vi "TLB Native Dynamic Events ver 0.07c.vi"() -> ()   [LabVIEW 2018]
uses:
  Labview Training Phase 2/Enum Controls/States for Action Engine.ctl
  Type def/TLB event states.ctl
  Type def/TLB MHL States.ctl
  <vilib>/Studica/Studica Toolkit/Background/I2C Channel.ctl
  <vilib>/Studica/Studica Toolkit/NavX/NavX.lvlib
  <vilib>/myRIO/Common/Instrument Driver Framework/myRIO v1.0/AI/typedefs/AI Channels Enum.ctl
  <vilib>/myRIO/Common/Instrument Driver Framework/myRIO v1.0/AI/typedefs/AI Channels List.ctl
  Type def/Type def.ctl
  Type def/Motor Control Cluster.ctl
  <vilib>/Studica/Studica Blackhawk/Blackhawk.lvlib
  <vilib>/Studica/Studica Toolkit/Background/Mxp Selection.ctl
  <vilib>/Studica/Studica Toolkit/Background/DIO Channel.ctl
  <vilib>/NI_Real-Time Target Support.lvlib
  <vilib>/ptbypt/NI_PtbyPt.lvlib
  <vilib>/addons/control/pid/NI_PID_pid.lvlib
  <vilib>/addons/control/pid/pid.llb/PID (DBL).vi
  Underlying VI's/Webcam FGV Low level ver/State control.ctl
  <vilib>/userdefined/High Color/IMAQdx.ctl
panel:
  out "Manual Zero Yaw":bool
  out "Cluster":T1
  out "Displacement":T2
  out "Fused Heading":dbl
  in  "error in (no error)":errorcluster
  in  "RED LED State":enum16{"OFF", "ON", "BLINK"}(ring)
  in  "GREEN LED State":enum16{"OFF", "ON", "BLINK"}(ring)
  in  "Red LED":bool
  in  "Green LED":bool
  in  "NavX Zero Yaw":bool
  out "Input state":i8
  out "Waveform Chart 2":dbl(graph)
  out "Waveform Chart":dbl(graph)
  in  "STOP":bool
  out "DIO 0":bool
  out "DIO 1":bool
  out "Limit Switch Array":bool[](array[boolean])
  out "error out":errorcluster
  out "L/R average":fxp<+,64,64>
  out "Right Ultrasonic":fxp<+,64,16>
  out "Left Ultrasonic":fxp<+,64,16>
  out "Right IR Sensor":dbl
  out "Left IR Sensor":dbl
  out "Object detection count":T3
  out "Camera error":errorcluster
  in  "Servo Angle":u8(slide) scale=0.0..180.0
  in  "On/Off":bool
  out "Error":errorcluster
  out "element":T4
  out "Action Queue Items":i32
  out "State Logic Queue Items":i32
  out "Action Queues items":string[](array[string])=["Hardware reset", "Software reset", ""]
  out "State logic":T5=enum."Task 2"
  out "Action State":string
  out "Yaw":dbl
  # "TLB FRAMEWORK STATUS"
  # "Camera Status Loop"
  # "Test Programme written by Calvin Loke    Dated: 28 Aug 2019\nTest Programme revised by Dr Alex See   Dated 30 Aug 2019\n\nProgramme version:   TLB Native Dynamic Events ver 0.04b.vi"
  # "Motor Control Loop"
  # "NAVX Control Loop"
  # "Blackhawk status"
  # "Sensor data"
  # "System Health Status Update"
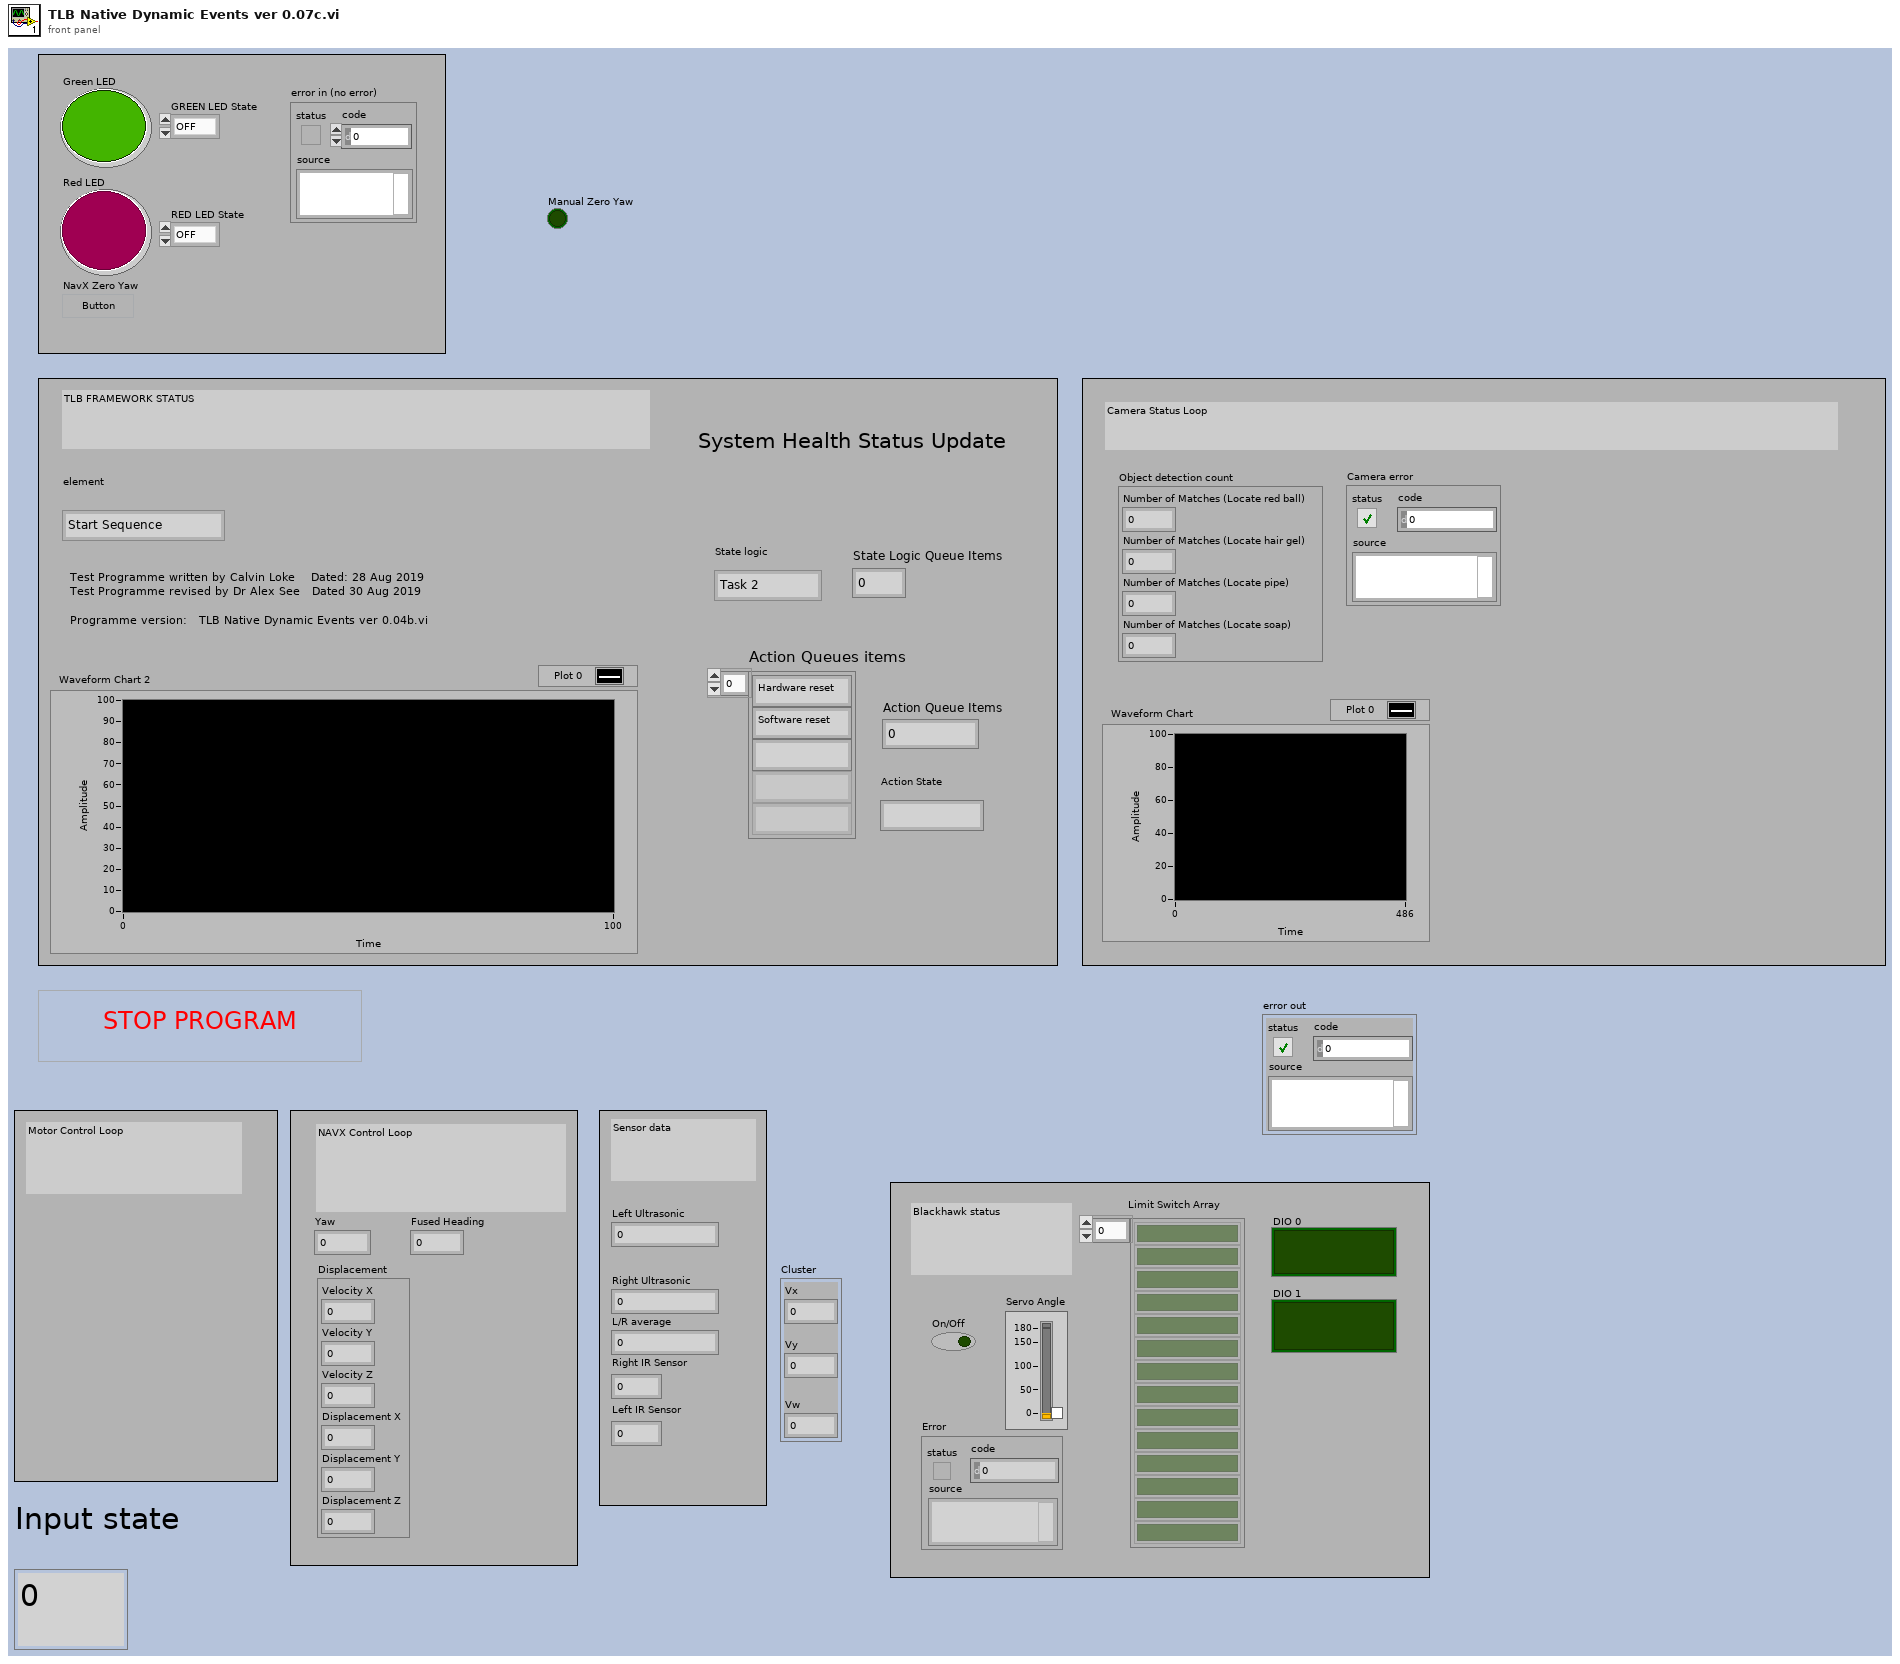
[diagram p1: front panel]
types:
  T1 = typedef "Motor Control Cluster.ctl" = cluster{"Vx":dbl, "Vy":dbl, "Vw":dbl}
  T2 = cluster{"Velocity X":dbl, "Velocity Y":dbl, "Velocity Z":dbl, "Displacement X":dbl, "Displacement Y":dbl, "Displacement Z":dbl}
  T3 = cluster{"Number of Matches (Locate red ball)":i32, "Number of Matches (Locate hair gel)":i32, "Number of Matches (Locate pipe)":i32, "Number of Matches (Locate soap)":i32}
  T4 = typedef "TLB event states.ctl" = enum16{"Start Sequence", "Exit", "Start Task 1", "Start Task 2", "Start Task 3", "Start Task 4", "Camera vision", "Wall follow mode", "Idle", "Start Drive Straight"}
  T5 = typedef "TLB MHL States.ctl" = enum16{"None", "Startup", "Idle", "Processing", "Shutdown", "Reset", "Task 1", "Task 2", "Task 3", "Task 4", "Task 4a", "Task 4b", "Task 4c", "Task 4d", "Task 4e", "Task 4f", "Task 4g", "Task 4h", "Acquire image", "Wall follow mode", "Autodrive", "Autodrive a"}
  T6 = typedef "States for Action Engine.ctl" = enum16{"Initialize", "Write", "Read"}
  T7 = typedef "DIO Channel.ctl" = enum16{"Not Connected", "A/DIO1", "A/DIO2", "A/DIO3", "A/DIO4", "A/DIO5", "A/DIO6", "A/DIO7", "A/DIO13", "B/DIO1", "B/DIO2", "B/DIO3", "B/DIO4", "B/DIO5", "B/DIO6", "B/DIO7", "B/DIO13", "C/DIO0", "C/DIO1", "C/DIO2", "C/DIO3", "C/DIO4", "C/DIO5", "C/DIO6", "C/DIO7"}
  T8 = typedef "Type def.ctl" = cluster{"Front Ultrasonic Obstruct":bool, "Left Ultrasonic Obstruct":bool, "Right Ultrasonic Obstruct ":bool}
  T9 = typedef "I2C Channel.ctl" = enum16{"Not Connected", "A", "B"}
  T10 = typedef "TLB MHL States.ctl" = enum16{"None", "Startup", "Idle", "Processing", "Shutdown", "Reset", "Task 1", "Task 2", "Task 3", "Task 4", "Task 4a", "Task 4b", "Task 4c", "Task 4d", "Task 4e", "Task 4f", "Task 4g", "Task 4h", "Acquire image", "Wall follow mode", "Drive Straight"}
  T11 = cluster{"proportional gain (Kc)":dbl, "integral time (Ti, min)":dbl, "derivative time (Td, min)":dbl}
  T12 = typedef "State control.ctl" = enum16{"Initialise", "Start camera", "Continuous Acquisition ", "Stop camera", "Dispose all"}
  T13 = typedef "IMAQdx.ctl" = refnum<k21>
  T14 = typedef "Mxp Selection.ctl" = enum16{"MXP A", "MXP B"}
  T15 = cluster{"xTargetSpeed":dbl, "yTargetSpeed":dbl, "wTargetSpeed":dbl}
  T16 = typedef "AI Channels List.ctl" = T17[]
  T17 = typedef "AI Channels Enum.ctl" = enum16{"Not Connected", "AudioIn/Left", "AudioIn/Right", "C/AI0", "C/AI1", "A/AI0", "A/AI1", "A/AI2", "A/AI3", "A/AI4", "A/AI5", "A/AI6", "A/AI7", "B/AI0", "B/AI1", "B/AI2", "B/AI3", "B/AI4", "B/AI5", "B/AI6", "B/AI7", "AI/AI0", "AI/AI1", "AI/AI2", "AI/AI3", "A/AI0 (DIFF)", "A/AI1 (DIFF)", "A/AI2 (DIFF)", "A/AI3 (DIFF)", "B/AI0 (DIFF)", "B/AI1 (DIFF)", "B/AI2 (DIFF)", "B/AI3 (DIFF)"}
  T18 = cluster{"DIO Channel":T7, "FPGA VI Reference Out":refnum<k20>}
  T19 = typedef "Analog Scaling Constants List.ctl" = T20[]
  T20 = typedef "Analog Scaling Constants.ctl" = cluster{"LSB Weight (Volts)":dbl, "Offset (Volts)":dbl, "Signed?":bool}
  T21 = cluster{"Scale Constants Array":T19, "FPGA Reference Out":refnum<k20>, "AI Channel":T16}
  T22 = cluster{"I2C Channel":T9, "FPGA VI Reference Out":refnum<k20>}
  T23 = typedef "NI_Real-Time Target Support.lvlib/RT CPU Load.ctl" = cluster{"Total (%)":dbl, "Time Critical (%)":dbl, "Timed Structures (%)":dbl, "High (%)":dbl, "Above Normal (%)":dbl, "Normal (%)":dbl, "Background (%)":dbl, "Idle (%)":dbl, "ISR (%)":dbl}
  T24 = cluster{"CPU loads[0]":T23, "CPU loads[1]":T23, "CPU loads[2]":T23, "CPU loads[3]":T23, "CPU loads[4]":T23, "CPU loads[5]":T23, "CPU loads[6]":T23, "CPU loads[7]":T23, "CPU loads[8]":T23}
  T25 = cluster{"I2C Ref Out":cluster{"I2C Channel":T9, "FPGA VI Reference Out":refnum<k20>}, "Connected":bool, "Slave Address (7-bit)":u8, "Registry":u8[]}
  T26 = cluster{"Yaw":dbl, "Roll":dbl, "Pitch":dbl, "Heading":dbl, "Fused Heading":dbl}
  T27 = typedef "IMAQ Image.ctl" = refnum<image>
  T28 = cluster{cluster{"xSpeed":dbl, "ySpeed":dbl, "wSpeed":dbl}, cluster{"xDistance":dbl, "yDistance":dbl, "wDistance":dbl}}
  T29 = cluster{"xDistance":dbl, "yDistance":dbl, "wDistance":dbl}
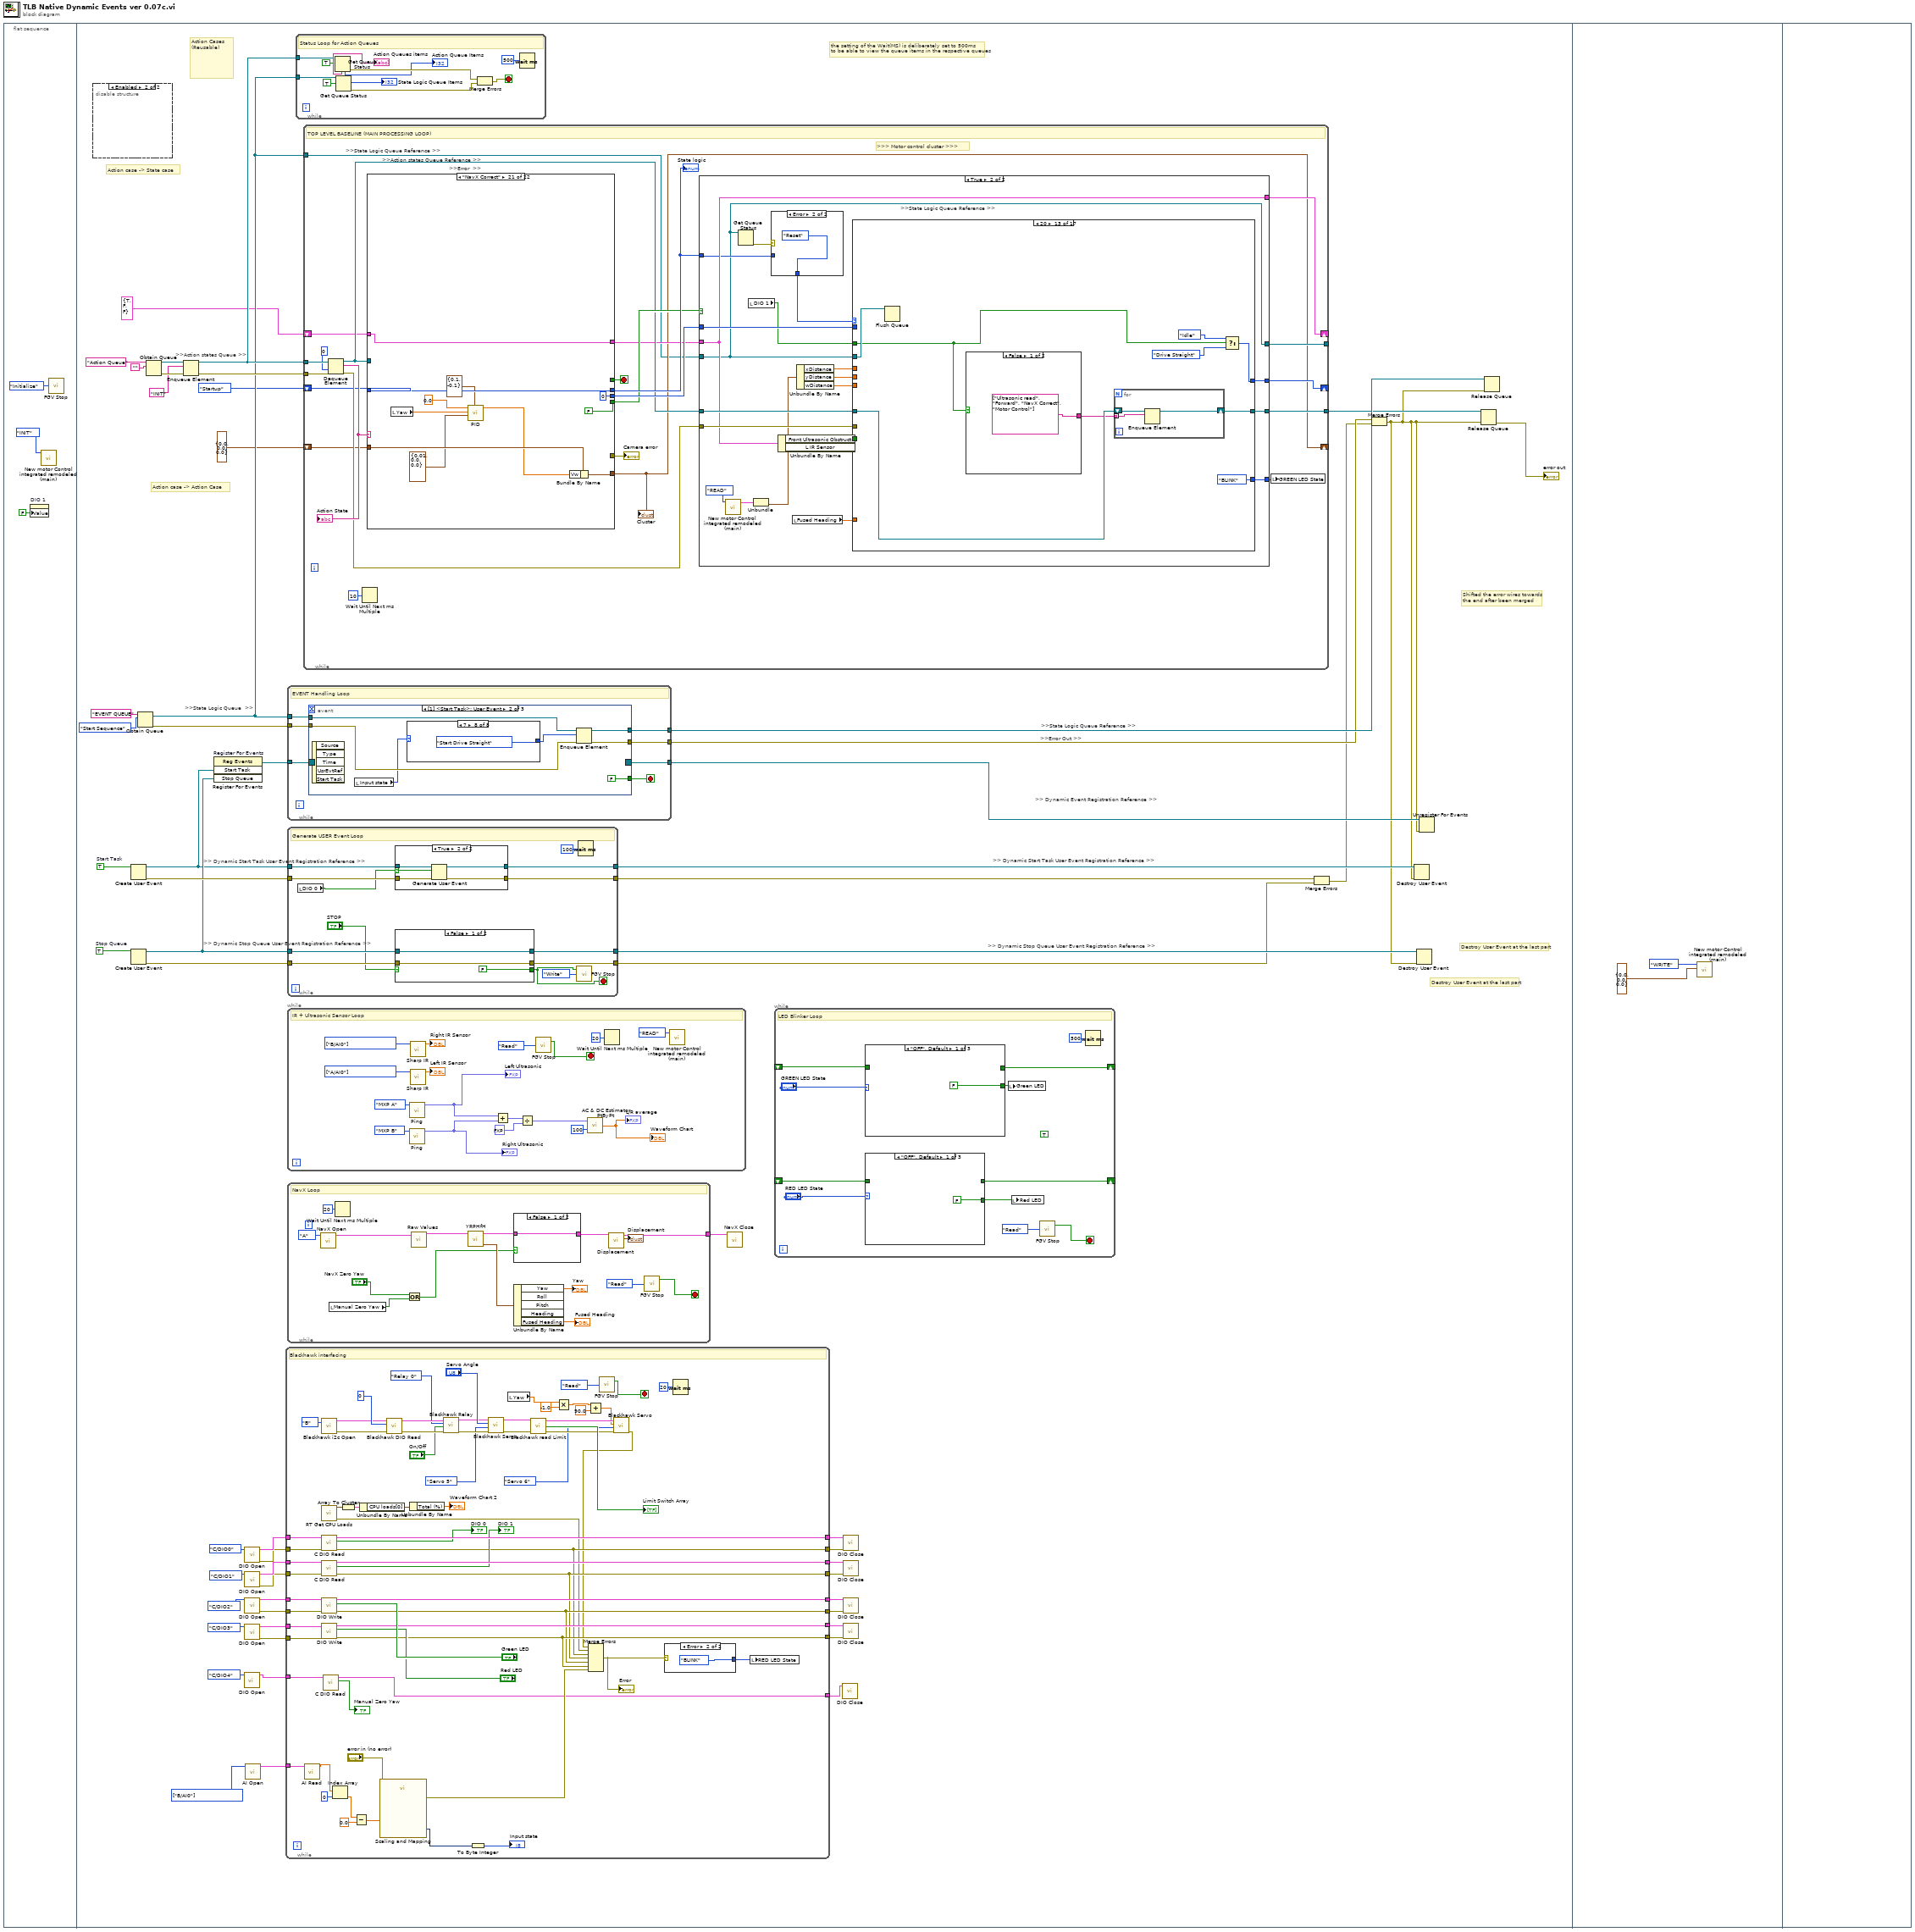
[diagram p0: block diagram]
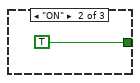
[diagram p2: hidden frame]
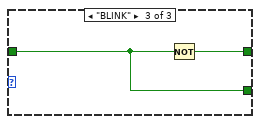
[diagram p3: hidden frame]
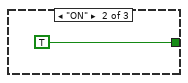
[diagram p4: hidden frame]
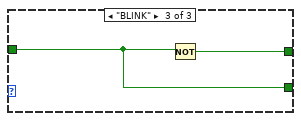
[diagram p5: hidden frame]
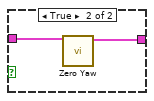
[diagram p6: hidden frame]
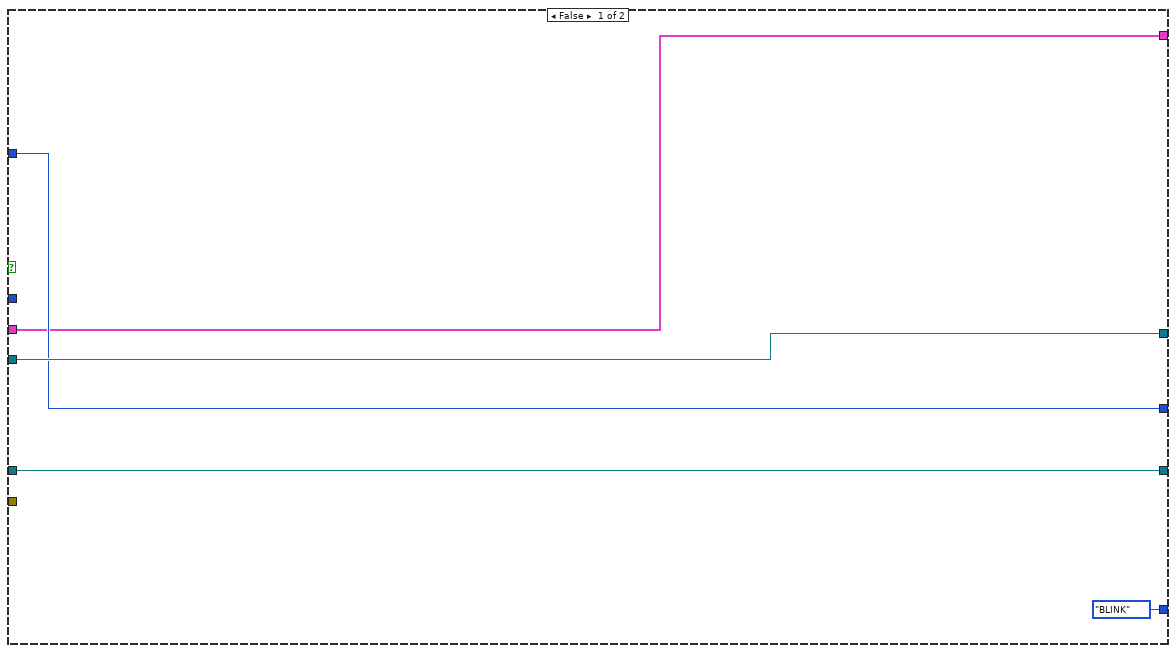
[diagram p7: hidden frame]
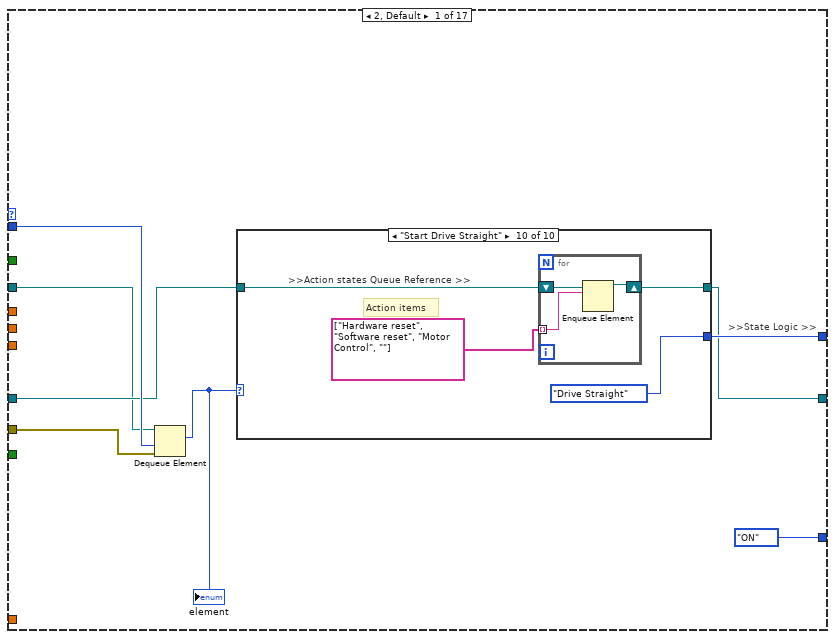
[diagram p9: hidden frame]
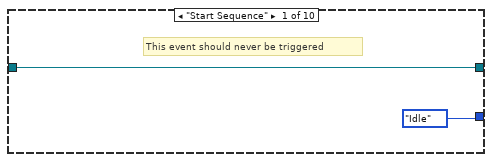
[diagram p10: hidden frame]
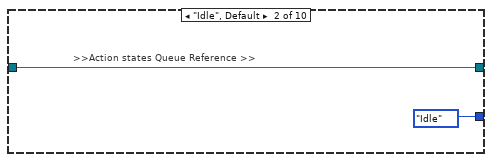
[diagram p11: hidden frame]
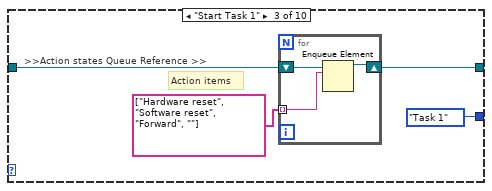
[diagram p12: hidden frame]
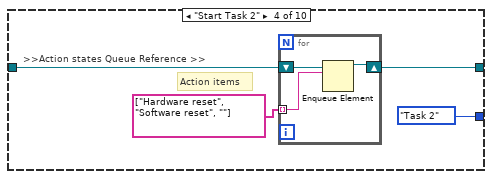
[diagram p13: hidden frame]
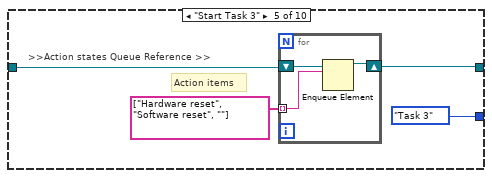
[diagram p14: hidden frame]
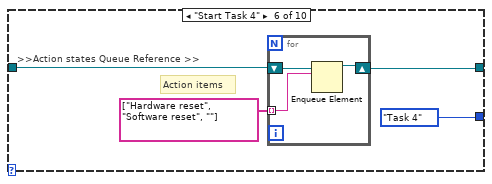
[diagram p15: hidden frame]
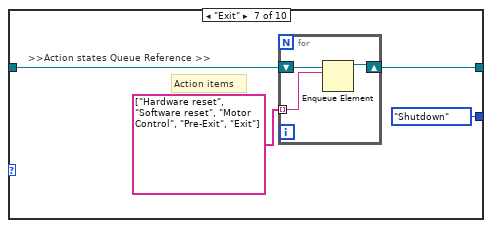
[diagram p16: hidden frame]
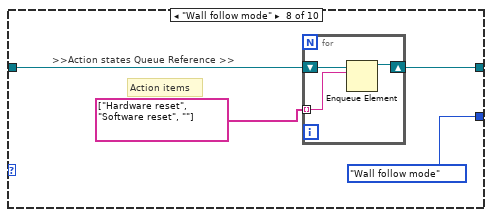
[diagram p17: hidden frame]
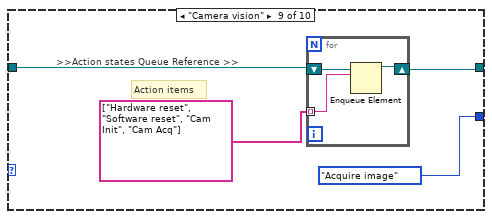
[diagram p18: hidden frame]
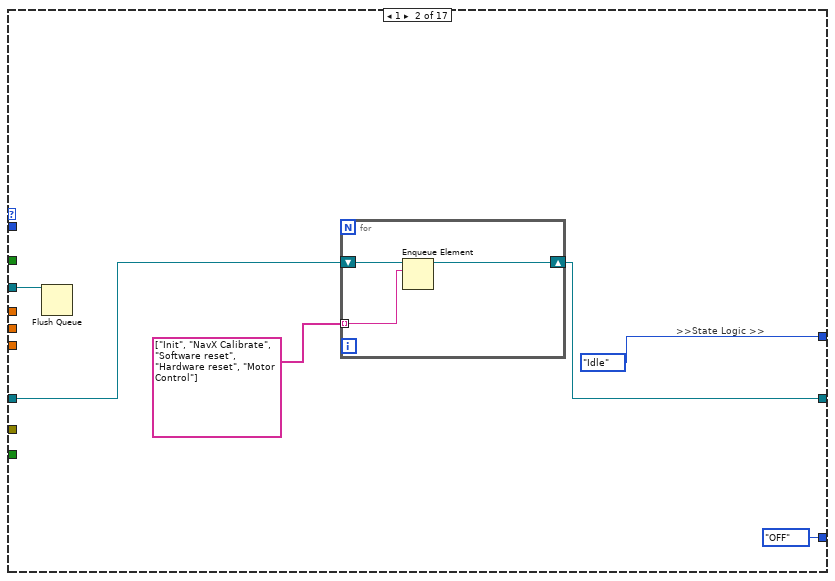
[diagram p19: hidden frame]
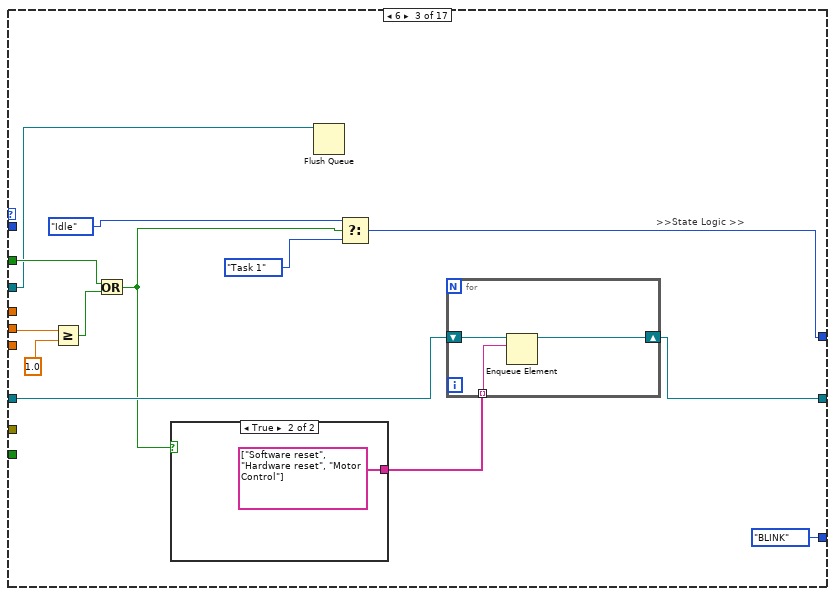
[diagram p20: hidden frame]
diagram:
  n1 = flat-sequence {
    frame #0 {
      n2 = property on="DIO 1" class="Bool (strict)"("Value"=FALSE ("DIO 1")) -> ()  [unwired: 2 in, 2 out]
      n3 = call "New motor Control integrated remodeled (main).vi"("States"=enum16{"RESET ENCODER", "WRITE", "READ", "INIT"}."INIT") -> ()  [unwired: 4 in, 2 out]
      n4 = call "FGV Stop.vi"("Init/Read/Write State"=States_for_Action_Engine."Initialize") -> ()  [unwired: 2 in, 2 out]
    }
    frame #1 {
      w12 = T16 [enum."B/AI0"] items=["Not Connected", "AudioIn/Left", "AudioIn/Right", "C/AI0", "C/AI1", "A/AI0", "A/AI1", "A/AI2", "A/AI3", "A/AI4", "A/AI5", "A/AI6", "A/AI7", "B/AI0", "B/AI1", "B/AI2", "B/AI3", "B/AI4", "B/AI5", "B/AI6", "B/AI7", "AI/AI0", "AI/AI1", "AI/AI2", "AI/AI3", "A/AI0 (DIFF)", "A/AI1 (DIFF)", "A/AI2 (DIFF)", "A/AI3 (DIFF)", "B/AI0 (DIFF)", "B/AI1 (DIFF)", "B/AI2 (DIFF)", "B/AI3 (DIFF)"] ("AI Channel")
      w61 = TRUE  # Stop Queue
      w60 = TRUE  # Start Task
      # "Action case -> Action Case"
      # "Action case -> State case"
      # "the setting of the Wait(MS) is deliberately set to 500ms\nto be able to view the queue items in the respective queues"
      # "Action Cases\n(Reusable)"
      # ">>Error Out >>"
      # ">> Dynamic Stop Queue User Event Registration Reference >>"
      # ">> Dynamic Start Task User Event Registration Reference >>"
      # ">> Dynamic Stop Queue User Event Registration Reference >>"
      # ">> Dynamic Start Task User Event Registration Reference >>"
      # ">> Dynamic Event Registration Reference >>"
      # ">>Action states Queue >>"
      # ">>State Logic Queue  >>"
      # ">>State Logic Queue Reference >>"
      # "Destroy User Event at the last part"
      # "Destroy User Event at the last part"
      # "Shifted the error wires towards\nthe end after been merged"
      n5 = disable-structure shown="Enabled" {
        frame Disabled {
          (unwired) variant
          (unwired) TRUE
          n6 = Variant To Data(type="") -> ()  [unwired: 2 in, 2 out]
        }
        frame Enabled {
        }
      }
      n7 = Create User Event(user event datatype=w60) -> (user event=w52:refnum<user-event>, error out=w57:errorcluster)  [unwired: 1 in]
      n8 = Create User Event(user event datatype=w61) -> (user event=w53:refnum<user-event>, error out=w56:errorcluster)  [unwired: 1 in]
      n9 = Obtain Queue(name (unnamed)="EVENT QUEUE", element data type=TLB_event_states."Start Sequence" ("Enum")) -> (queue out=w37:refnum<queue>, error out=w43:errorcluster)  [unwired: 3 in, 1 out]
      n10 = Obtain Queue(name (unnamed)="Action Queue", element data type="") -> (queue out=w46:refnum<queue>, error out=w42:errorcluster)  [unwired: 3 in, 1 out]
      n11 = Enqueue Element(queue=w46, element="INIT", error in (no error)=w42) -> (queue out=w38:refnum<queue>, error out=w41:errorcluster)  [unwired: 1 in, 1 out]
      n12 = register-events "Register For Events"(w52, w53) -> (reference out=w51:refnum<event-registration>)  [unwired: 2 in, 1 out]
      n13 = call <vilib>:"DIO Open.vi"("DIO Channel"=DIO_Channel."C/DIO4") -> ("DIO Info Out"=w6:T18)  [unwired: 9 in, 1 out]
      n14 = call <vilib>:"DIO Open.vi"("DIO Channel"=DIO_Channel."C/DIO0") -> ("error out"=w22:errorcluster, "DIO Info Out"=w28:T18)  [unwired: 9 in]
      n15 = call <vilib>:"DIO Open.vi"("DIO Channel"=DIO_Channel."C/DIO1") -> ("error out"=w20:errorcluster, "DIO Info Out"=w24:T18)  [unwired: 9 in]
      n16 = call <vilib>:"DIO Open.vi"("DIO Channel"=DIO_Channel."C/DIO2") -> ("error out"=w10:errorcluster, "DIO Info Out"=w16:T18)  [unwired: 9 in]
      n17 = call <vilib>:"DIO Open.vi"("DIO Channel"=DIO_Channel."C/DIO3") -> ("error out"=w8:errorcluster, "DIO Info Out"=w15:T18)  [unwired: 9 in]
      n18 = call <vilib>:"AI Open.vi"("AI Channel"=w12) -> ("Analog Info"=w11:T21)  [unwired: 9 in, 1 out]
      n19 = while {
        tunnel: w28 -> [w749]
        tunnel: [w748] -> w27
        tunnel: w24 -> [w747]
        tunnel: [w746] -> w23
        tunnel: w22 -> [w745]
        tunnel: [w714] -> w21
        tunnel: w20 -> [w744]
        tunnel: [w715] -> w19
        tunnel: w16 -> [w738]
        tunnel: w15 -> [w737]
        tunnel: [w734] -> w14
        tunnel: [w733] -> w13
        tunnel: w11 -> [w732]
        tunnel: w10 -> [w725]
        tunnel: [w716] -> w9
        tunnel: w8 -> [w724]
        tunnel: [w717] -> w7
        tunnel: w6 -> [w705]
        tunnel: [w704] -> w4
        stop <- w762 stop-if-true
        # "Blackhawk interfacing"
        n20 = call <vilib>:"AI Read.vi"("Analog Info"=w732) -> ("Array"=w728:dbl[])  [unwired: 9 in, 1 out]
        n21 = call <vilib>:"Blackhawk i2c Open.vi"("I2C Channel"=I2C_Channel."B") -> ("I2C Ref Out"=w740:T22, "error out"=w739:errorcluster)  [unwired: 2 in]
        n22 = call <vilib>:"RT Get CPU Loads.vi"() -> ("error out"=w713:errorcluster, "CPU loads"=w719:T23[])  [unwired: 10 in]
        n23 = call <vilib>:"C DIO Read.vi"("error in (no error)"=w745, "DIO Info In in"=w749) -> ("error out"=w714:errorcluster, "IN"=→"DIO 0":bool, "DIO Info In out"=w748:T18)  [unwired: 7 in]
        n24 = call <vilib>:"C DIO Read.vi"("error in (no error)"=w744, "DIO Info In in"=w747) -> ("error out"=w715:errorcluster, "IN"=→"DIO 1":bool, "DIO Info In out"=w746:T18)  [unwired: 7 in]
        n25 = call <vilib>:"DIO Write.vi"("error in (no error)"=w725, "Input"="Green LED", "DIO Info In"=w738) -> ("error out"=w716:errorcluster, "DIO Info Out"=w734:T18)  [unwired: 7 in]
        n26 = call <vilib>:"DIO Write.vi"("error in (no error)"=w724, "Input"="Red LED", "DIO Info In"=w737) -> ("error out"=w717:errorcluster, "DIO Info Out"=w733:T18)  [unwired: 7 in]
        n27 = call <vilib>:"C DIO Read.vi"("DIO Info In in"=w705) -> ("IN"=→"Manual Zero Yaw":bool, "DIO Info In out"=w704:T18)  [unwired: 8 in, 1 out]
        n28 = Index Array(array=w728, index=0) -> (element=w730:dbl)
        n29 = Array To Cluster(array=w719) -> (cluster=w720:T24)
        n30 = Subtract(x=w730, y=0.0) -> (x-y=w731:dbl)
        n31 = Unbundle By Name(w720) -> ("CPU loads[0]"=w721:T23)
        n32 = call "Scaling and Mapping"("error in (no error)"="error in (no error)", "Signals"=w731) -> ("error out"=w718:errorcluster, "Scaled Signals"=w726:dynamicdata)  [unwired: 8 in]
        n33 = call <vilib>:"Blackhawk DIO Read.vi"("I2C Ref In"=w740, "PIN"=u8 0, "error in (no error)"=w739) -> ("I2C Ref Out"=w760:T22, "error out"=w761:errorcluster)  [unwired: 3 in, 1 out]
        n34 = Unbundle By Name(w721) -> ("Total (%)"=→"Waveform Chart 2":dbl)
        n35 = call <vilib>:"Blackhawk Relay.vi"("error in (no error)"=w761, "On/Off"="On/Off", "Relay"=enum8{"Relay 0", "Relay 1", "Relay 2"}."Relay 0", "I2C Ref In"=w760) -> ("error out"=w757:errorcluster, "I2C Ref Out"=w754:T22)  [unwired: 6 in]
        n36 = To Byte Integer(number=w726) -> (8bit integer=→"Input state":i8)
        n37 = call <vilib>:"Blackhawk Servo.vi"("error in (no error)"=w757, "Servo Select"=enum16{"Servo 5", "Servo 6"}."Servo 5", "Servo Angle"="Servo Angle", "I2C Ref In"=w754) -> ("error out"=w752:errorcluster, "I2C Ref Out"=w751:T22)  [unwired: 6 in]
        n38 = local read "Yaw"() -> (w699:dbl)
        n39 = call <vilib>:"Blackhawk read Limit.vi"("error in (no error)"=w752, "I2C Ref In"=w751) -> ("error out"=w709:errorcluster, "Limit Switch Array"=→"Limit Switch Array":bool[], "I2C Ref Out"=w707:T22)  [unwired: 1 in]
        n40 = Multiply(x=w699, y=-1.0) -> (x*y=w700:dbl)
        n41 = Add(x=w700, y=90.0) -> (x+y=w701:dbl)
        n42 = call "FGV Stop.vi"("Init/Read/Write State"=States_for_Action_Engine."Read") -> ("Output node"=w762:bool)  [unwired: 2 in, 1 out]
        n43 = call <vilib>:"Blackhawk Servo.vi"("error in (no error)"=w709, "Servo Select"=enum16{"Servo 5", "Servo 6"}."Servo 6", "Servo Angle"=w701, "I2C Ref In"=w707) -> ("error out"=w708:errorcluster)  [unwired: 6 in, 1 out]
        n44 = Merge Errors(w708, w713, w714, w715, w716, w717, w718) -> (w712:errorcluster)
        "Error" <- w712
        n45 = case shown="Error" w712 {
          tunnel: [enum16{"OFF", "ON", "BLINK"}."OFF" ("RED LED State") enum16{"OFF", "ON", "BLINK"}."BLINK" ("RED LED State")] -> w723
          frame No Error {
          }
          frame Error {
          }
        }
        n46 = Wait (ms)(milliseconds to wait=u32 20) -> ()  [unwired: 1 out]
        n47 = local write "RED LED State"(w723) -> ()
      }
      n48 = while {
        tunnel: w51 -> [w642]
        tunnel: [w641] -> w50
        tunnel: w37 -> [w639]
        tunnel: [w638] -> w49
        tunnel: w43 -> [w637]
        tunnel: [w636] -> w40
        stop <- w640 stop-if-true
        # "EVENT Handling Loop"
        n49 = event shown="[1] <Start Task>: User Event" {
          selector: w642 -> [_ _ _]
          dyn-events: [_ _ _] -> w641
          timeout: _ -> [_ _ _]
          tunnel: [FALSE FALSE w669] -> w640
          tunnel: w639 -> [w647 w654 w667]
          tunnel: [w646 w653 w668] -> w638
          tunnel: w637 -> [w644 w652 w665]
          tunnel: [w643 w651 w664] -> w636
          event Timeout {
            n50 = event-data() -> ()  [unwired: 1 in, 3 out]
            n51 = Enqueue Element(queue=w647, element=TLB_event_states."Idle" ("Enum"), error in (no error)=w644) -> (queue out=w646:refnum<queue>, error out=w643:errorcluster)  [unwired: 1 in, 1 out]
          }
          event User Event {
            n52 = event-data() -> ()  [unwired: 1 in, 5 out]
            n53 = local read "Input state"() -> (w650:i8)
            n54 = case shown="7" w650 {
              tunnel: [TLB_event_states."Idle" ("Enum") TLB_event_states."Start Task 1" ("Enum") TLB_event_states."Start Task 2" ("Enum") TLB_event_states."Start Task 3" ("Enum") TLB_event_states."Start Task 4" ("Enum") TLB_event_states."Wall follow mode" ("Enum") TLB_event_states."Camera vision" ("Enum") TLB_event_states."Start Drive Straight" ("Enum")] -> w649
              frame 0 {
              }
              frame 1 {
              }
              frame 2 {
              }
              frame 3, Default {
              }
              frame 4 {
              }
              frame 5 {
              }
              frame 6 {
              }
              frame 7 {
              }
            }
            n55 = Enqueue Element(queue=w654, element=w649, error in (no error)=w652) -> (queue out=w653:refnum<queue>, error out=w651:errorcluster)  [unwired: 1 in, 1 out]
          }
          event User Event {
            n56 = event-data() -> ("Stop Queue"=w669:bool)  [unwired: 1 in, 4 out]
            n57 = Enqueue Element At Opposite End(queue=w667, element=TLB_event_states."Exit" ("Enum"), error in (no error)=w665) -> (queue out=w668:refnum<queue>, error out=w664:errorcluster)  [unwired: 1 in, 1 out]
          }
        }
      }
      n58 = while {
        tunnel: w52 -> [w681]
        tunnel: w53 -> [w680]
        tunnel: [w679] -> w59
        tunnel: [w678] -> w58
        tunnel: w57 -> [w677]
        tunnel: [w676] -> w55
        tunnel: w56 -> [w675]
        tunnel: [w674] -> w54
        stop <- w672 stop-if-true
        # "Generate USER Event Loop"
        n59 = local read "DIO 0"() -> (w671:bool)
        n60 = case shown="True" w671 {
          selector: w671 -> [_ w693]
          tunnel: w681 -> [w692 w697]
          tunnel: [w692 w696] -> w678
          tunnel: w677 -> [w691 w695]
          tunnel: [w691 w694] -> w676
          frame False {
          }
          frame True {
            n61 = Generate User Event(user event=w697, event data cluster=w693, error in=w695) -> (user event out=w696:refnum<user-event>, error out=w694:errorcluster)  [unwired: 1 in]
          }
        }
        n62 = case shown="False" "STOP" {
          selector: "STOP" -> [_ w686]
          tunnel: w680 -> [w685 w690]
          tunnel: [w685 w689] -> w679
          tunnel: w675 -> [w684 w688]
          tunnel: [w684 w687] -> w674
          tunnel: [FALSE w686] -> w672
          frame False {
          }
          frame True {
            n63 = Generate User Event(user event=w690, event data cluster=w686, error in=w688) -> (user event out=w689:refnum<user-event>, error out=w687:errorcluster)  [unwired: 1 in]
          }
        }
        n64 = call "FGV Stop.vi"("Init/Read/Write State"=States_for_Action_Engine."Write", "Input Node"=w672) -> ()  [unwired: 1 in, 2 out]
        n65 = Wait (ms)(milliseconds to wait=u32 100) -> ()  [unwired: 1 out]
      }
      n66 = while {
        stop <- w618 stop-if-true
        w623 = T16 [enum."A/AI0"] items=["Not Connected", "AudioIn/Left", "AudioIn/Right", "C/AI0", "C/AI1", "A/AI0", "A/AI1", "A/AI2", "A/AI3", "A/AI4", "A/AI5", "A/AI6", "A/AI7", "B/AI0", "B/AI1", "B/AI2", "B/AI3", "B/AI4", "B/AI5", "B/AI6", "B/AI7", "AI/AI0", "AI/AI1", "AI/AI2", "AI/AI3", "A/AI0 (DIFF)", "A/AI1 (DIFF)", "A/AI2 (DIFF)", "A/AI3 (DIFF)", "B/AI0 (DIFF)", "B/AI1 (DIFF)", "B/AI2 (DIFF)", "B/AI3 (DIFF)"] ("AI Channel")
        w624 = T16 [enum."B/AI0"] items=["Not Connected", "AudioIn/Left", "AudioIn/Right", "C/AI0", "C/AI1", "A/AI0", "A/AI1", "A/AI2", "A/AI3", "A/AI4", "A/AI5", "A/AI6", "A/AI7", "B/AI0", "B/AI1", "B/AI2", "B/AI3", "B/AI4", "B/AI5", "B/AI6", "B/AI7", "AI/AI0", "AI/AI1", "AI/AI2", "AI/AI3", "A/AI0 (DIFF)", "A/AI1 (DIFF)", "A/AI2 (DIFF)", "A/AI3 (DIFF)", "B/AI0 (DIFF)", "B/AI1 (DIFF)", "B/AI2 (DIFF)", "B/AI3 (DIFF)"] ("AI Channel")
        # "IR + Ultrasonic Sensor Loop"
        n67 = call <vilib>:"Ping.vi"("Mxp Side"=Mxp_Selection."MXP B") -> ("CM"=w612:fxp<+,64,16>)  [unwired: 8 in, 2 out]
        "Right Ultrasonic" <- w612
        n68 = call <vilib>:"Ping.vi"("Mxp Side"=Mxp_Selection."MXP A") -> ("CM"=w613:fxp<+,64,16>)  [unwired: 8 in, 2 out]
        "Left Ultrasonic" <- w613
        n69 = call <vilib>:"Sharp IR.vi"("AI Channel"=w624) -> ("Sharp IR Distance"=→"Right IR Sensor":dbl)  [unwired: 8 in, 2 out]
        n70 = call <vilib>:"Sharp IR.vi"("AI Channel"=w623) -> ("Sharp IR Distance"=→"Left IR Sensor":dbl)  [unwired: 8 in, 2 out]
        n71 = Add(x=w613, y=w612) -> (x+y=w615:fxp<+,64,17>)
        n72 = Divide(x=w615, y=fxp<+,64,17> 2.0) -> (x/y=w611:fxp<+,64,64>)
        n73 = call "FGV Stop.vi"("Init/Read/Write State"=States_for_Action_Engine."Read") -> ("Output node"=w618:bool)  [unwired: 2 in, 1 out]
        n74 = call <vilib>:"AC & DC Estimator PtByPt.vi"("signal"=w611, "sample length"=100) -> ("DC estimate (V)"=→"L/R average" →"Waveform Chart":dbl)  [unwired: 1 in, 2 out]
        n75 = Wait Until Next ms Multiple(millisecond multiple=u32 20) -> ()  [unwired: 1 out]
        n76 = call "New motor Control integrated remodeled (main).vi"("States"=enum16{"RESET ENCODER", "WRITE", "READ", "INIT"}."READ") -> ()  [unwired: 4 in, 2 out]
      }
      n77 = while {
        tunnel: [w87] -> w29
        stop <- w95 stop-if-true
        # "NavX Loop"
        n78 = call <vilib>:"NavX Open.vi"("I2C Channel"=I2C_Channel."A") -> ("NavX Info"=w89:T25)  [unwired: 9 in, 1 out]
        n79 = local read "Manual Zero Yaw"() -> (w82:bool)
        n80 = Wait Until Next ms Multiple(millisecond multiple=u32 20) -> ()  [unwired: 1 out]
        n81 = Or(x="NavX Zero Yaw", y=w82) -> (x .or. y?=w83:bool)
        n82 = call <vilib>:"Raw Values.vi"("NavX Info In"=w89) -> ("NavX Info Out"=w92:T25)  [unwired: 8 in, 1 out]
        n83 = call <vilib>:"YRPHfH.vi"("NavX Info In"=w92) -> ("YRPHfH"=w93:T26, "NavX Info Out"=w91:T25)  [unwired: 3 in]
        n84 = case shown="False" w83 {
          tunnel: [w97 w99] -> w88
          tunnel: w91 -> [w97 w98]
          frame False {
          }
          frame True {
            n85 = call <vilib>:"Zero Yaw.vi"("NavX Info In"=w98) -> ("NavX Info Out"=w99:T25)  [unwired: 10 in]
          }
        }
        n86 = Unbundle By Name(w93) -> ("Yaw"=→"Yaw":dbl, "Fused Heading"=→"Fused Heading":dbl)  [unwired: 3 out]
        n87 = call <vilib>:"Displacement.vi"("NavX Info In"=w88) -> ("Displacement"=→"Displacement":T2, "NavX Info Out"=w87:T25)  [unwired: 9 in]
        n88 = call "FGV Stop.vi"("Init/Read/Write State"=States_for_Action_Engine."Read") -> ("Output node"=w95:bool)  [unwired: 2 in, 1 out]
      }
      n89 = while {
        tunnel: w38 -> [w633]
        tunnel: w37 -> [w630]
        stop <- w627 stop-if-true
        # "Status Loop for Action Queues"
        n90 = Get Queue Status(queue=w633, return elements? (F)=TRUE) -> (error out=w629:errorcluster, # elements in queue=→"Action Queue Items":i32, elements=→"Action Queues items":string[])  [unwired: 1 in, 5 out]
        n91 = Get Queue Status(queue=w630, return elements? (F)=TRUE) -> (# pending remove=→"State Logic Queue Items":i32, error out=w628:errorcluster)  [unwired: 1 in, 6 out]
        n92 = Merge Errors(w629, w628) -> (w627:errorcluster)
        n93 = Wait (ms)(milliseconds to wait=u32 500) -> ()  [unwired: 1 out]
      }
      n94 = while {
        tunnel: w37 -> [w103]
        shift-right: [w116] -> _
        shift-left: TLB_MHL_States."Startup" ("Enum") -> [w110]
        tunnel: w38 -> [w121]
        tunnel: w41 -> [w119]
        tunnel: [w118] -> _
        tunnel: [w117] -> w32
        shift-right: [w107] -> _
        shift-left: T8 {"Front Ultrasonic Obstruct"=TRUE, "Left Ultrasonic Obstruct"=FALSE, "Right Ultrasonic Obstruct "=FALSE} -> [w109]
        shift-right: [w105] -> _
        shift-left: T1 {"Vx"=0.0, "Vy"=0.0, "Vw"=0.0} -> [w106]
        stop <- w101 stop-if-true
        # ">>> Motor control cluster >>>"
        # ">>Error  >>"
        # ">>Action states Queue Reference >>"
        # ">>State Logic Queue Reference >>"
        # "TOP LEVEL BASELINE (MAIN PROCESSING LOOP)"
        n95 = Dequeue Element(queue=w121, timeout in ms (-1)=0, error in (no error)=w119) -> (queue out=w111:refnum<queue>, element=w120:string, error out=w112:errorcluster)  [unwired: 1 out]
        "Action State" <- w120
        n96 = Wait Until Next ms Multiple(millisecond multiple=u32 10) -> ()  [unwired: 1 out]
        n97 = case shown="\"NavX Correct\"" w120 {
          tunnel: [w422 w434 w441 w449 w458 w466 w472 w482 w489 w495 w505 w515 TLB_MHL_States."Shutdown" ("Enum") w526 w536 w540 w555 w567 w575 w589 w598 w604] -> w122
          tunnel: [w426 0 0 0 0 0 0 0 0 0 0 0 0 0 0 0 0 0 0 0 0 0] -> w115
          tunnel: [TRUE FALSE FALSE FALSE FALSE FALSE FALSE FALSE FALSE FALSE FALSE FALSE FALSE FALSE FALSE FALSE FALSE FALSE FALSE FALSE FALSE FALSE] -> w114
          tunnel: w111 -> [_ _ _ _ _ _ _ _ _ _ _ _ _ _ _ _ _ _ _ _ _ _]
          tunnel: w110 -> [w422 w434 w441 w449 w458 w466 w472 w482 w489 w495 w505 w515 _ w526 w536 w540 w555 w567 w575 w589 w598 w604]
          tunnel: w109 -> [w424 w431 w438 w446 w454 w462 w470 w478 w486 w496 w502 w511 w518 w527 w535 w543 w556 w568 w574 w585 w596 w606]
          tunnel: [w424 w431 w438 w446 w454 w462 w470 w478 w486 w496 w501 w511 w518 w527 w532 w542 w556 w568 w574 w585 w596 w606] -> w108
          tunnel: w106 -> [w423 w430 w436 w444 w452 w461 w468 w477 w484 w492 w499 w510 w517 w523 w529 w537 w551 w566 w578 w586 w599 w605]
          tunnel: [w423 w430 w437 w445 w453 w460 w469 w476 w485 w492 w499 w508 w517 w523 w529 w537 w552 w566 w578 w586 w600 w605] -> w105
          tunnel: [_ _ _ _ _ _ _ _ _ _ _ _ _ _ _ _ _ w557 w570 w579 _ _] -> w104
          tunnel: [_ _ _ _ _ _ _ _ _ _ _ _ TRUE _ _ _ _ _ _ _ _ _] -> w101
          frame "No action", Default {
            n98 = case shown="1, Default" w422 {
              tunnel: [0 100] -> w426
              frame 1, Default {
              }
              frame 2 {
              }
            }
            n99 = local write "NavX Zero Yaw"(FALSE ("NavX Zero Yaw")) -> ()
          }
          frame "Init" {
            # ">>State Logic  >>"
            n100 = local write "Servo Angle"(u8 90 ("Servo Angle")) -> ()
          }
          frame "Forward" {
            n101 = local write "NavX Zero Yaw"(FALSE ("NavX Zero Yaw")) -> ()
            n102 = Bundle By Name(cluster=w436, "Vy"=0.6) -> (w437:T1)
          }
          frame "Reverse" {
            n103 = local write "NavX Zero Yaw"(FALSE ("NavX Zero Yaw")) -> ()
            n104 = Bundle By Name(cluster=w444, "Vy"=-0.6) -> (w445:T1)
          }
          frame "Right" {
            n105 = local write "NavX Zero Yaw"(FALSE ("NavX Zero Yaw")) -> ()
            n106 = Bundle By Name(cluster=w452, "Vx"=0.6) -> (w453:T1)
          }
          frame "Left" {
            n107 = Bundle By Name(cluster=w461, "Vx"=-0.6) -> (w460:T1)
            n108 = local write "NavX Zero Yaw"(FALSE ("NavX Zero Yaw")) -> ()
          }
          frame "Rotate CW" {
            n109 = local write "NavX Zero Yaw"(FALSE ("NavX Zero Yaw")) -> ()
            n110 = Bundle By Name(cluster=w468, "Vw"=-0.3) -> (w469:T1)
          }
          frame "Rotate ACW" {
            n111 = local write "NavX Zero Yaw"(FALSE ("NavX Zero Yaw")) -> ()
            n112 = Bundle By Name(cluster=w477, "Vw"=0.15) -> (w476:T1)
          }
          frame "Stop" {
            w483 = 0.0
            n113 = local write "NavX Zero Yaw"(FALSE ("NavX Zero Yaw")) -> ()
            n114 = Bundle By Name(cluster=w484, "Vx"=w483, "Vy"=w483, "Vw"=w483) -> (w485:T1)
          }
          frame "Motor control" {
            n115 = call "New motor Control integrated remodeled (main).vi"("States"=enum16{"RESET ENCODER", "WRITE", "READ", "INIT"}."WRITE", "Target Speed"=w492) -> ()  [unwired: 3 in, 2 out]
          }
          frame "Software reset" {
            w500 = FALSE ("NavX Zero Yaw")
            n116 = Wait (ms)(milliseconds to wait=u32 20) -> ()  [unwired: 1 out]
            n117 = local write "NavX Zero Yaw"(w500) -> ()
            n118 = Bundle By Name(cluster=w502, "Front Ultrasonic Obstruct"=w500, "L IR Sensor"=0.0) -> (w501:T8)
          }
          frame "Hardware reset" {
            w509 = 0.0
            n119 = Wait (ms)(milliseconds to wait=u32 100) -> ()  [unwired: 1 out]
            n120 = local write "NavX Zero Yaw"(TRUE ("NavX Zero Yaw")) -> ()
            n121 = call "New motor Control integrated remodeled (main).vi"("States"=enum16{"RESET ENCODER", "WRITE", "READ", "INIT"}."RESET ENCODER") -> ()  [unwired: 4 in, 2 out]
            n122 = Bundle By Name(cluster=w510, "Vx"=w509, "Vy"=w509, "Vw"=w509) -> (w508:T1)
          }
          frame "Exit" {
          }
          frame "Pre-Exit" {
            n123 = call "New motor Control integrated remodeled (main).vi"("States"=enum16{"RESET ENCODER", "WRITE", "READ", "INIT"}."INIT") -> ()  [unwired: 4 in, 2 out]
          }
          frame "Ultrasonic read" {
            # "Object detection"
            n124 = local read "L/R average"() -> (w528:fxp<+,64,64>)
            n125 = Less Or Equal?(x=w528, y=35.0) -> (x <= y?=w530:bool)
            n126 = Bundle By Name(cluster=w535, "Front Ultrasonic Obstruct"=w530) -> (w532:T8)
          }
          frame "IR Sensor Read" {
            n127 = local read "Left IR Sensor"() -> (w541:dbl)
            n128 = Bundle By Name(cluster=w543, "L IR Sensor"=w541) -> (w542:T8)
          }
          frame "Calculate" {
            n129 = Unbundle By Name(w556) -> ("L IR Sensor"=w548:dbl)
            n130 = call-poly <vilib>:"PID.vi"("output range"=cluster{"output high":dbl, "output low":dbl} {"output high"=0.3, "output low"=-0.3}, "PID gains"=T11 {"proportional gain (Kc)"=0.01, "integral time (Ti, min)"=0.0, "derivative time (Td, min)"=0.0}, "process variable"=w548, "setpoint"=20.0) -> ("output"=w545:dbl)  [unwired: 6 in, 1 out]
            n131 = Negate(x=w545) -> (-x=w544:dbl)
            n132 = Bundle By Name(cluster=w551, "Vy"=0.2, "Vw"=w544) -> (w552:T1)
          }
          frame "Cam Init" {
            n133 = call "Low-Level Grab.vi"("States"=State_control."Initialise", "Session In"=T13 "cam1") -> ("error out"=w558:errorcluster, "Session Out"=w559:T13)  [unwired: 7 in, 1 out]
            n134 = call "Low-Level Grab.vi"("error in (no error)"=w558, "States"=State_control."Start camera", "Session In"=w559) -> ("error out"=w557:errorcluster)  [unwired: 6 in, 2 out]
            n135 = local write "Servo Angle"(u8 170 ("Servo Angle")) -> ()
          }
          frame "Cam Acq" {
            n136 = call "Low-Level Grab.vi"("States"=State_control."Continuous Acquisition ") -> ("error out"=w571:errorcluster, "Image Out"=w572:T27)  [unwired: 8 in, 1 out]
            n137 = call "All object detection ver2.vi"("Image In"=w572, "error in"=w571) -> ("Object detection count"=→"Object detection count":T3, "error out"=w570:errorcluster)  [unwired: 1 out]
          }
          frame "Cam Exit" {
            n138 = call "Low-Level Grab.vi"("States"=State_control."Stop camera") -> ("error out"=w580:errorcluster, "Session Out"=w582:T13)  [unwired: 8 in, 1 out]
            n139 = call "Low-Level Grab.vi"("error in (no error)"=w580, "States"=State_control."Dispose all", "Session In"=w582) -> ("error out"=w579:errorcluster)  [unwired: 6 in, 2 out]
            n140 = local write "Servo Angle"(u8 90 ("Servo Angle")) -> ()
          }
          frame "NavX Correct" {
            n141 = local read "Yaw"() -> (w590:dbl)
            n142 = call-poly <vilib>:"PID.vi"("output range"=cluster{"output high":dbl, "output low":dbl} {"output high"=0.1, "output low"=-0.1}, "PID gains"=T11 {"proportional gain (Kc)"=0.01, "integral time (Ti, min)"=0.0, "derivative time (Td, min)"=0.0}, "process variable"=w590, "setpoint"=0.0 ("y")) -> ("output"=w591:dbl)  [unwired: 6 in, 1 out]
            n143 = Bundle By Name(cluster=w599, "Vw"=w591) -> (w600:T1)
          }
          frame "NavX Calibrate" {
            # "Adds a 15 second delay to the startup process \nfor the NavX to calibrate"
            n144 = Wait (ms)(milliseconds to wait=u32 15000) -> ()  [unwired: 1 out]
          }
        }
        "State logic" <- w122
        "Camera error" <- w104
        "Cluster" <- w105
        n145 = case shown="True" w114 {
          tunnel: w122 -> [w126 w132]
          tunnel: w103 -> [w127 w131]
          tunnel: w111 -> [w125 w147]
          tunnel: [w127 w131] -> w118
          tunnel: [w125 w146] -> w117
          tunnel: [w126 w145] -> w116
          tunnel: w112 -> [_ w144]
          tunnel: w115 -> [_ w143]
          tunnel: w108 -> [w124 w137]
          tunnel: [w124 w137] -> w107
          tunnel: [enum16{"OFF", "ON", "BLINK"}."BLINK" ("GREEN LED State") w128] -> w100
          frame False {
          }
          frame True {
            # ">>State Logic Queue Reference >>"
            n146 = call "New motor Control integrated remodeled (main).vi"("States"=enum16{"RESET ENCODER", "WRITE", "READ", "INIT"}."READ") -> ("Speed and distance cluster"=w136:T28)  [unwired: 4 in, 1 out]
            n147 = Get Queue Status(queue=w131) -> (error out=w130:errorcluster)  [unwired: 2 in, 7 out]
            n148 = local read "DIO 1"() -> (w129:bool)
            n149 = Unbundle(w136) -> (w135:T29)  [unwired: 1 out]
            n150 = case shown="Error" w130 {
              tunnel: [w148 TLB_MHL_States."Reset" ("Enum")] -> w133
              tunnel: w132 -> [w148 _]
              frame No Error {
              }
              frame Error {
              }
            }
            n151 = Unbundle By Name(w137) -> ("Front Ultrasonic Obstruct"=w138:bool)  [unwired: 1 out]
            n152 = local read "Fused Heading"() -> (w139:dbl)
            n153 = Unbundle By Name(w135) -> ("xDistance"=w140:dbl, "yDistance"=w142:dbl, "wDistance"=w141:dbl)
            n154 = case shown="20" w133 {
              tunnel: w131 -> [w151 w218 w228 w246 w265 w281 w295 w311 w327 w344 _ w368 w384 w396 _ _ _]
              tunnel: w147 -> [w153 w221 w235 w250 w274 w285 w301 w318 w333 w350 w361 w371 w385 w400 w409 w413 w419]
              tunnel: [w152 w220 w234 w251 w273 w286 w300 w317 w332 w349 w360 w372 w386 w399 w409 w412 w419] -> w146
              tunnel: [w156 TLB_MHL_States."Idle" ("Enum") w237 w252 w270 w289 w303 w316 w334 w348 TLB_MHL_States."Shutdown" ("Enum") w374 w387 w398 TLB_MHL_States."Reset" ("Enum") TLB_MHL_States."Shutdown" ("Enum") TLB_MHL_States."Reset" ("Enum")] -> w145
              tunnel: w144 -> [w154 _ _ _ _ _ _ _ _ _ _ _ _ _ _ _ _]
              tunnel: w143 -> [w155 _ _ _ _ _ _ _ _ _ _ _ _ _ _ _ _]
              tunnel: w129 -> [_ _ w232 w249 w268 _ _ _ _ w347 _ w369 w382 w397 _ _ _]
              tunnel: w142 -> [_ _ w229 _ _ _ _ w313 _ _ _ _ _ _ _ _ _]
              tunnel: w141 -> [_ _ _ _ _ _ _ _ _ _ _ _ _ _ _ _ _]
              tunnel: w140 -> [_ _ _ _ _ _ w297 _ w329 _ _ _ _ _ _ _ _]
              tunnel: w139 -> [_ _ _ _ w264 _ _ _ _ _ _ _ _ _ _ _ _]
              tunnel: w138 -> [_ _ _ w247 _ w283 _ _ _ w346 _ _ _ _ _ _ _]
              tunnel: [enum16{"OFF", "ON", "BLINK"}."ON" ("GREEN LED State") enum16{"OFF", "ON", "BLINK"}."OFF" ("GREEN LED State") enum16{"OFF", "ON", "BLINK"}."BLINK" ("GREEN LED State") enum16{"OFF", "ON", "BLINK"}."BLINK" ("GREEN LED State") enum16{"OFF", "ON", "BLINK"}."BLINK" ("GREEN LED State") enum16{"OFF", "ON", "BLINK"}."BLINK" ("GREEN LED State") enum16{"OFF", "ON", "BLINK"}."BLINK" ("GREEN LED State") enum16{"OFF", "ON", "BLINK"}."BLINK" ("GREEN LED State") enum16{"OFF", "ON", "BLINK"}."BLINK" ("GREEN LED State") enum16{"OFF", "ON", "BLINK"}."BLINK" ("GREEN LED State") enum16{"OFF", "ON", "BLINK"}."OFF" ("GREEN LED State") enum16{"OFF", "ON", "BLINK"}."BLINK" ("GREEN LED State") enum16{"OFF", "ON", "BLINK"}."BLINK" ("GREEN LED State") enum16{"OFF", "ON", "BLINK"}."BLINK" ("GREEN LED State") _ enum16{"OFF", "ON", "BLINK"}."OFF" ("GREEN LED State") _] -> w128
              frame 2, Default {
                # ">>State Logic >>"
                n155 = Dequeue Element(queue=w151, timeout in ms (-1)=w155, error in (no error)=w154) -> (element=w157:T4)  [unwired: 3 out]
                "element" <- w157
                n156 = case shown="\"Start Drive Straight\"" w157 {
                  tunnel: [TLB_MHL_States."Idle" ("Enum") TLB_MHL_States."Idle" ("Enum") TLB_MHL_States."Task 1" ("Enum") TLB_MHL_States."Task 2" ("Enum") TLB_MHL_States."Task 3" ("Enum") TLB_MHL_States."Task 4" ("Enum") TLB_MHL_States."Shutdown" ("Enum") TLB_MHL_States."Wall follow mode" ("Enum") TLB_MHL_States."Acquire image" ("Enum") TLB_MHL_States."Drive Straight" ("Enum")] -> w156
                  tunnel: [w159 w160 w164 w169 w178 w184 w190 w197 w205 w212] -> w152
                  tunnel: w153 -> [w159 w160 w162 w170 w179 w185 w191 w198 w206 w213]
                  frame "Start Sequence" {
                    # "This event should never be triggered"
                  }
                  frame "Idle", Default {
                    # ">>Action states Queue Reference >>"
                  }
                  frame "Start Task 1" {
                    # ">>Action states Queue Reference >>"
                    # "Action items"
                    n157 = for {
                      shift-right: [w168] -> w164
                      shift-left: w162 -> [w167]
                      tunnel: string[] ["Hardware reset", "Software reset", "Forward", ""] -> [w166] mode=indexing
                      n158 = Enqueue Element(queue=w167, element=w166) -> (queue out=w168:refnum<queue>)  [unwired: 2 in, 2 out]
                    }
                  }
                  frame "Start Task 2" {
                    # ">>Action states Queue Reference >>"
                    # "Action items"
                    n159 = for {
                      shift-right: [w175] -> w169
                      shift-left: w170 -> [w174]
                      tunnel: string[] ["Hardware reset", "Software reset", ""] -> [w173] mode=indexing
                      n160 = Enqueue Element(queue=w174, element=w173) -> (queue out=w175:refnum<queue>)  [unwired: 2 in, 2 out]
                    }
                  }
                  frame "Start Task 3" {
                    # ">>Action states Queue Reference >>"
                    # "Action items"
                    n161 = for {
                      shift-right: [w182] -> w178
                      shift-left: w179 -> [w181]
                      tunnel: string[] ["Hardware reset", "Software reset", ""] -> [w180] mode=indexing
                      n162 = Enqueue Element(queue=w181, element=w180) -> (queue out=w182:refnum<queue>)  [unwired: 2 in, 2 out]
                    }
                  }
                  frame "Start Task 4" {
                    # ">>Action states Queue Reference >>"
                    # "Action items"
                    n163 = for {
                      shift-right: [w189] -> w184
                      shift-left: w185 -> [w188]
                      tunnel: string[] ["Hardware reset", "Software reset", ""] -> [w187] mode=indexing
                      n164 = Enqueue Element(queue=w188, element=w187) -> (queue out=w189:refnum<queue>)  [unwired: 2 in, 2 out]
                    }
                  }
                  frame "Exit" {
                    # ">>Action states Queue Reference >>"
                    # "Action items"
                    n165 = for {
                      shift-right: [w196] -> w190
                      shift-left: w191 -> [w195]
                      tunnel: string[] ["Hardware reset", "Software reset", "Motor Control", "Pre-Exit", "Exit"] -> [w194] mode=indexing
                      n166 = Enqueue Element(queue=w195, element=w194) -> (queue out=w196:refnum<queue>)  [unwired: 2 in, 2 out]
                    }
                  }
                  frame "Wall follow mode" {
                    # ">>Action states Queue Reference >>"
                    # "Action items"
                    n167 = for {
                      shift-right: [w203] -> w197
                      shift-left: w198 -> [w202]
                      tunnel: string[] ["Hardware reset", "Software reset", ""] -> [w201] mode=indexing
                      n168 = Enqueue Element(queue=w202, element=w201) -> (queue out=w203:refnum<queue>)  [unwired: 2 in, 2 out]
                    }
                  }
                  frame "Camera vision" {
                    # ">>Action states Queue Reference >>"
                    # "Action items"
                    n169 = for {
                      shift-right: [w210] -> w205
                      shift-left: w206 -> [w209]
                      tunnel: string[] ["Hardware reset", "Software reset", "Cam Init", "Cam Acq"] -> [w208] mode=indexing
                      n170 = Enqueue Element(queue=w209, element=w208) -> (queue out=w210:refnum<queue>)  [unwired: 2 in, 2 out]
                    }
                  }
                  frame "Start Drive Straight" {
                    # ">>Action states Queue Reference >>"
                    # "Action items"
                    n171 = for {
                      shift-right: [w217] -> w212
                      shift-left: w213 -> [w216]
                      tunnel: string[] ["Hardware reset", "Software reset", "Motor Control", ""] -> [w215] mode=indexing
                      n172 = Enqueue Element(queue=w216, element=w215) -> (queue out=w217:refnum<queue>)  [unwired: 2 in, 2 out]
                    }
                  }
                }
              }
              frame 1 {
                # ">>State Logic >>"
                n173 = Flush Queue(queue=w218) -> ()  [unwired: 1 in, 3 out]
                n174 = for {
                  shift-right: [w225] -> w220
                  shift-left: w221 -> [w226]
                  tunnel: string[] ["Init", "NavX Calibrate", "Software reset", "Hardware reset", "Motor Control"] -> [w224] mode=indexing
                  n175 = Enqueue Element(queue=w226, element=w224) -> (queue out=w225:refnum<queue>)  [unwired: 2 in, 2 out]
                }
              }
              frame 6 {
                # ">>State Logic >>"
                n176 = Greater Or Equal?(x=w229, y=1.0) -> (x >= y?=w230:bool)
                n177 = Or(x=w232, y=w230) -> (x .or. y?=w233:bool)
                n178 = case shown="True" w233 {
                  tunnel: [string[] ["Forward", "Motor Control", ""] string[] ["Software reset", "Hardware reset", "Motor Control"]] -> w236
                  frame False {
                  }
                  frame True {
                  }
                }
                n179 = Flush Queue(queue=w228) -> ()  [unwired: 1 in, 3 out]
                n180 = Select(t=TLB_MHL_States."Idle" ("Enum"), s=w233, f=TLB_MHL_States."Task 1" ("Enum")) -> (s? t:f=w237:T5)
                n181 = for {
                  shift-right: [w243] -> w234
                  shift-left: w235 -> [w244]
                  tunnel: w236 -> [w242] mode=indexing
                  n182 = Enqueue Element(queue=w244, element=w242) -> (queue out=w243:refnum<queue>)  [unwired: 2 in, 2 out]
                }
              }
              frame 7 {
                # ">>State Logic >>"
                n183 = Flush Queue(queue=w246) -> ()  [unwired: 1 in, 3 out]
                n184 = case shown="True" w249 {
                  tunnel: [w256 string[] ["Hardware reset", "Software reset", "Motor control"]] -> w248
                  tunnel: w247 -> [w255 _]
                  frame False {
                    n185 = case shown="False" w255 {
                      tunnel: [string[] ["Stop", "Ultrasonic read", "Motor Control"] string[] ["Reverse", "Ultrasonic read", "Motor control"]] -> w256
                      frame False {
                      }
                      frame True {
                      }
                    }
                  }
                  frame True {
                  }
                }
                n186 = Select(t=TLB_MHL_States."Idle" ("Enum"), s=w249, f=TLB_MHL_States."Task 2" ("Enum")) -> (s? t:f=w252:T5)
                n187 = for {
                  shift-right: [w261] -> w251
                  shift-left: w250 -> [w262]
                  tunnel: w248 -> [w260] mode=indexing
                  n188 = Enqueue Element(queue=w262, element=w260) -> (queue out=w261:refnum<queue>)  [unwired: 2 in, 2 out]
                }
              }
              frame 8 {
                n189 = Greater Or Equal?(x=w264, y=360.0) -> (x >= y?=w267:bool)
                n190 = Flush Queue(queue=w265) -> ()  [unwired: 1 in, 3 out]
                n191 = Or(x=w267, y=w268) -> (x .or. y?=w269:bool)
                n192 = case shown="False" w269 {
                  tunnel: [string[] ["Rotate CW", "Motor Control"] string[] ["Software reset", "Hardware reset", "Motor Control"]] -> w275
                  frame False {
                  }
                  frame True {
                  }
                }
                n193 = for {
                  shift-right: [w277] -> w273
                  shift-left: w274 -> [w278]
                  tunnel: w275 -> [w276] mode=indexing
                  n194 = Enqueue Element(queue=w278, element=w276) -> (queue out=w277:refnum<queue>)  [unwired: 2 in, 2 out]
                }
                n195 = Select(t=TLB_MHL_States."Idle" ("Enum"), s=w269, f=TLB_MHL_States."Task 3" ("Enum")) -> (s? t:f=w270:T5)
              }
              frame 9 {
                n196 = Flush Queue(queue=w281) -> ()  [unwired: 1 in, 3 out]
                n197 = case shown="True" w283 {
                  tunnel: [string[] ["Forward", "Ultrasonic read", "Motor Control"] string[] ["Stop", "Hardware reset", "Software reset", "Motor Control"]] -> w284
                  frame False {
                  }
                  frame True {
                  }
                }
                n198 = for {
                  shift-right: [w293] -> w286
                  shift-left: w285 -> [w294]
                  tunnel: w284 -> [w292] mode=indexing
                  n199 = Enqueue Element(queue=w294, element=w292) -> (queue out=w293:refnum<queue>)  [unwired: 2 in, 2 out]
                }
                n200 = Select(t=TLB_MHL_States."Task 4a" ("Enum"), s=w283, f=TLB_MHL_States."Task 4" ("Enum")) -> (s? t:f=w289:T5)
              }
              frame 10 {
                n201 = Greater Or Equal?(x=w297, y=0.5) -> (x >= y?=w299:bool)
                n202 = Flush Queue(queue=w295) -> ()  [unwired: 1 in, 3 out]
                n203 = case shown="True" w299 {
                  tunnel: [string[] ["Right", "Motor Control"] string[] ["Stop", "Hardware reset", "Software reset", "Motor Control"]] -> w302
                  frame False {
                  }
                  frame True {
                  }
                }
                n204 = for {
                  shift-right: [w309] -> w300
                  shift-left: w301 -> [w310]
                  tunnel: w302 -> [w308] mode=indexing
                  n205 = Enqueue Element(queue=w310, element=w308) -> (queue out=w309:refnum<queue>)  [unwired: 2 in, 2 out]
                }
                n206 = Select(t=TLB_MHL_States."Task 4b" ("Enum"), s=w299, f=TLB_MHL_States."Task 4a" ("Enum")) -> (s? t:f=w303:T5)
              }
              frame 11 {
                n207 = Flush Queue(queue=w311) -> ()  [unwired: 1 in, 3 out]
                n208 = Greater Or Equal?(x=w313, y=0.75) -> (x >= y?=w314:bool)
                n209 = case shown="False" w314 {
                  tunnel: [string[] ["Forward", "Motor control"] string[] ["Stop", "Hardware reset", "Software reset"]] -> w319
                  frame False {
                  }
                  frame True {
                  }
                }
                n210 = for {
                  shift-right: [w325] -> w317
                  shift-left: w318 -> [w326]
                  tunnel: w319 -> [w324] mode=indexing
                  n211 = Enqueue Element(queue=w326, element=w324) -> (queue out=w325:refnum<queue>)  [unwired: 2 in, 2 out]
                }
                n212 = Select(t=TLB_MHL_States."Task 4c" ("Enum"), s=w314, f=TLB_MHL_States."Task 4b" ("Enum")) -> (s? t:f=w316:T5)
              }
              frame 12 {
                n213 = Flush Queue(queue=w327) -> ()  [unwired: 1 in, 3 out]
                n214 = Less Or Equal?(x=w329, y=-0.65) -> (x <= y?=w330:bool)
                n215 = case shown="False" w330 {
                  tunnel: [string[] ["Left", "Motor Control"] string[] ["Stop", "Hardware reset", "Software reset", "Motor Control"]] -> w335
                  frame False {
                  }
                  frame True {
                  }
                }
                n216 = for {
                  shift-right: [w341] -> w332
                  shift-left: w333 -> [w342]
                  tunnel: w335 -> [w340] mode=indexing
                  n217 = Enqueue Element(queue=w342, element=w340) -> (queue out=w341:refnum<queue>)  [unwired: 2 in, 2 out]
                }
                n218 = Select(t=TLB_MHL_States."Task 4d" ("Enum"), s=w330, f=TLB_MHL_States."Task 4c" ("Enum")) -> (s? t:f=w334:T5)
              }
              frame 13 {
                n219 = Flush Queue(queue=w344) -> ()  [unwired: 1 in, 3 out]
                n220 = Or(x=w347, y=w346) -> (x .or. y?=w345:bool)
                n221 = case shown="True" w345 {
                  tunnel: [string[] ["Forward", "Ultrasonic Read", "Motor Control"] string[] ["Stop", "Hardware reset", "Software reset", "Motor Control"]] -> w351
                  frame False {
                  }
                  frame True {
                  }
                }
                n222 = for {
                  shift-right: [w357] -> w349
                  shift-left: w350 -> [w358]
                  tunnel: w351 -> [w356] mode=indexing
                  n223 = Enqueue Element(queue=w358, element=w356) -> (queue out=w357:refnum<queue>)  [unwired: 2 in, 2 out]
                }
                n224 = Select(t=TLB_MHL_States."Idle" ("Enum"), s=w345, f=TLB_MHL_States."Task 4d" ("Enum")) -> (s? t:f=w348:T5)
              }
              frame 5 {
                n225 = for {
                  shift-right: [w365] -> w360
                  shift-left: w361 -> [w366]
                  tunnel: string[] ["Software reset", "Hardware reset", "Motor Control"] -> [w364] mode=indexing
                  n226 = Enqueue Element(queue=w366, element=w364) -> (queue out=w365:refnum<queue>)  [unwired: 2 in, 2 out]
                }
              }
              frame 19 {
                n227 = Flush Queue(queue=w368) -> ()  [unwired: 1 in, 3 out]
                n228 = case shown="False" w369 {
                  tunnel: [string[] ["IR Sensor Read", "Calculate", "Forward", "Motor Control"] string[] ["Hardware reset", "Software reset", "Motor Control"]] -> w370
                  frame False {
                  }
                  frame True {
                  }
                }
                n229 = for {
                  shift-right: [w379] -> w372
                  shift-left: w371 -> [w380]
                  tunnel: w370 -> [w378] mode=indexing
                  n230 = Enqueue Element(queue=w380, element=w378) -> (queue out=w379:refnum<queue>)  [unwired: 2 in, 2 out]
                }
                n231 = Select(t=TLB_MHL_States."Idle" ("Enum"), s=w369, f=TLB_MHL_States."Wall follow mode" ("Enum")) -> (s? t:f=w374:T5)
              }
              frame 20 {
                n232 = Flush Queue(queue=w384) -> ()  [unwired: 1 in, 3 out]
                n233 = case shown="False" w382 {
                  tunnel: [string[] ["Ultrasonic read", "Forward", "NavX Correct", "Motor Control"] string[] ["Hardware reset", "Software reset", "Motor Control", ""]] -> w381
                  frame False {
                  }
                  frame True {
                  }
                }
                n234 = for {
                  shift-right: [w393] -> w386
                  shift-left: w385 -> [w394]
                  tunnel: w381 -> [w392] mode=indexing
                  n235 = Enqueue Element(queue=w394, element=w392) -> (queue out=w393:refnum<queue>)  [unwired: 2 in, 2 out]
                }
                n236 = Select(t=TLB_MHL_States."Idle" ("Enum"), s=w382, f=TLB_MHL_States."Drive Straight" ("Enum")) -> (s? t:f=w387:u16)
              }
              frame 18 {
                n237 = Flush Queue(queue=w396) -> ()  [unwired: 1 in, 3 out]
                n238 = case shown="True" w397 {
                  tunnel: [string[] ["Cam Acq"] string[] ["Hardware reset", "Software reset", "Cam Exit", ""]] -> w401
                  frame False {
                  }
                  frame True {
                  }
                }
                n239 = for {
                  shift-right: [w407] -> w399
                  shift-left: w400 -> [w408]
                  tunnel: w401 -> [w406] mode=indexing
                  n240 = Enqueue Element(queue=w408, element=w406) -> (queue out=w407:refnum<queue>)  [unwired: 2 in, 2 out]
                }
                n241 = Select(t=TLB_MHL_States."Idle" ("Enum"), s=w397, f=TLB_MHL_States."Acquire image" ("Enum")) -> (s? t:f=w398:T5)
              }
              frame 3 {
              }
              frame 4 {
                # ">>State Logic >>"
                n242 = for {
                  shift-right: [w417] -> w412
                  shift-left: w413 -> [w418]
                  tunnel: string[] ["Software reset", "Hardware reset", "Motor Control", "Cam Exit", "Pre-Exit", "Exit"] -> [w416] mode=indexing
                  n243 = Enqueue Element(queue=w418, element=w416) -> (queue out=w417:refnum<queue>)  [unwired: 2 in, 2 out]
                }
              }
              frame 0 {
              }
            }
          }
        }
        n244 = local write "GREEN LED State"(w100) -> ()
      }
      n245 = call <vilib>:"NavX Close.vi"("NavX Info In"=w29) -> ()  [unwired: 10 in, 1 out]
      n246 = while {
        shift-right: [w64] -> _
        shift-left: _ -> [w65]
        shift-right: [w63] -> _
        shift-left: _ -> [w62]
        stop <- w71 stop-if-true
        (unwired) TRUE
        # "LED Blinker Loop"
        n247 = case shown="\"OFF\", Default" "GREEN LED State" {
          tunnel: [FALSE TRUE w79] -> w67
          tunnel: w65 -> [_ _ w79]
          tunnel: [_ _ w80] -> w64
          frame "OFF", Default {
          }
          frame "ON" {
          }
          frame "BLINK" {
            n248 = Not(x=w79) -> (.not. x?=w80:bool)
          }
        }
        n249 = case shown="\"OFF\", Default" "RED LED State" {
          tunnel: [FALSE TRUE w75] -> w66
          tunnel: [_ _ w76] -> w63
          tunnel: w62 -> [_ _ w75]
          frame "OFF", Default {
          }
          frame "ON" {
          }
          frame "BLINK" {
            n250 = Not(x=w75) -> (.not. x?=w76:bool)
          }
        }
        n251 = local write "Green LED"(w67) -> ()
        n252 = local write "Red LED"(w66) -> ()
        n253 = call "FGV Stop.vi"("Init/Read/Write State"=States_for_Action_Engine."Read") -> ("Output node"=w71:bool)  [unwired: 2 in, 1 out]
        n254 = Wait (ms)(milliseconds to wait=u32 500) -> ()  [unwired: 1 out]
      }
      n255 = call <vilib>:"DIO Close.vi"("DIO Info In"=w4) -> ()  [unwired: 10 in, 1 out]
      n256 = call <vilib>:"DIO Close.vi"("error in (no error)"=w21, "DIO Info In"=w27) -> ()  [unwired: 9 in, 1 out]
      n257 = call <vilib>:"DIO Close.vi"("error in (no error)"=w19, "DIO Info In"=w23) -> ()  [unwired: 9 in, 1 out]
      n258 = call <vilib>:"DIO Close.vi"("error in (no error)"=w9, "DIO Info In"=w14) -> ()  [unwired: 9 in, 1 out]
      n259 = call <vilib>:"DIO Close.vi"("error in (no error)"=w7, "DIO Info In"=w13) -> ()  [unwired: 9 in, 1 out]
      n260 = Merge Errors "Merge Errors"(w55, w54) -> (w36:errorcluster)
      n261 = Merge Errors(w40, w36) -> (w30:errorcluster)
      n262 = Destroy User Event(user event=w58, error in=w30) -> ()  [unwired: 1 out]
      n263 = Destroy User Event(user event=w59, error in=w30) -> ()  [unwired: 1 out]
      n264 = Unregister For Events(event registration refnum=w50, error in=w30) -> ()  [unwired: 1 out]
      n265 = Release Queue(queue=w32, error in (no error)=w30) -> (error out=→"error out":errorcluster)  [unwired: 1 in, 2 out]
      n266 = Release Queue(queue=w49, error in (no error)=w30) -> ()  [unwired: 1 in, 3 out]
    }
    frame #2 {
      n267 = call "New motor Control integrated remodeled (main).vi"("States"=enum16{"RESET ENCODER", "WRITE", "READ", "INIT"}."WRITE", "Target Speed"=T15 {"xTargetSpeed"=0.0, "yTargetSpeed"=0.0, "wTargetSpeed"=0.0}) -> ()  [unwired: 3 in, 2 out]
    }
    frame #3 {
    }
  }
